vi "UpdatePanels.vi"(8 "error in (no error)":errorcluster, 10 "Engine in":refnum<class "Engine.lvclass">, 11 "BounceDemo in":refnum<class "BounceDemo.lvclass">) -> (0 "error out":errorcluster, 2 "Engine out":refnum<class "Engine.lvclass">, 3 "Game out":refnum<class "BounceDemo.lvclass">)   [LabVIEW 2019, in "RT_Game.lvlib" / "BounceDemo.lvclass"]
uses:
  BounceDemo.lvclass
  C:/Users/FreshBob/Dropbox/VIs/myRIO_GameConsole/RT/RT_Game/Bouncer/Bouncer.lvclass
  Engine/Engine.lvclass
  Bouncer/Bouncer.lvclass/Bouncer.ctl
  Bouncer/Read Panel1.vi
  Bouncer/Read Panel2.vi
  Bouncer/Read Ball.vi
  Bouncer/Write Panel1.vi
  Bouncer/Write Panel2.vi
  BouncePanel/BouncePanel.lvclass
  PongBall/PongBall.lvclass
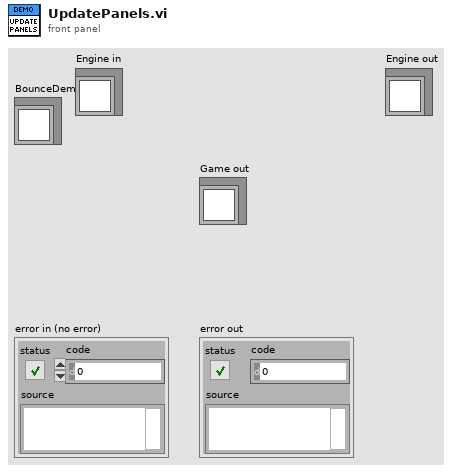
[diagram p1: front panel]
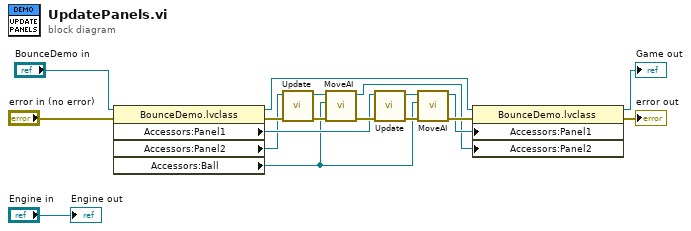
[diagram p0: block diagram]
diagram:
  n1 = property class="BounceDemo.lvclass"(reference="BounceDemo in", error in="error in (no error)") -> (reference out=w9:refnum<class "BounceDemo.lvclass">, error out=w15:errorcluster, "Accessors:Panel1"=w12:refnum<class "BouncePanel.lvclass">, "Accessors:Panel2"=w11:refnum<class "BouncePanel.lvclass">, "Accessors:Ball"=w4:refnum<class "PongBall.lvclass">)
  n2 = call-dynamic "Update.vi"("error in (no error)"=w15, "GameObject in"=w11) -> ("error out"=w6:errorcluster, "GameObject out"=w5:refnum<class "BouncePanel.lvclass">)  [unwired: 8 in]
  n3 = call-dynamic "MoveAI.vi"("error in (no error)"=w6, "Ball"=w4, "BouncePanel in"=w5) -> ("error out"=w16:errorcluster, "BouncePanel out"=w7:refnum<class "BouncePanel.lvclass">)  [unwired: 7 in]
  n4 = call-dynamic "Update.vi"("error in (no error)"=w16, "GameObject in"=w12) -> ("error out"=w18:errorcluster, "GameObject out"=w17:refnum<class "BouncePanel.lvclass">)  [unwired: 8 in]
  n5 = call-dynamic "MoveAI.vi"("error in (no error)"=w18, "Ball"=w4, "BouncePanel in"=w17) -> ("error out"=w10:errorcluster, "BouncePanel out"=w8:refnum<class "BouncePanel.lvclass">)  [unwired: 7 in]
  n6 = property class="BounceDemo.lvclass"(reference=w9, error in=w10, "Accessors:Panel1"=w8, "Accessors:Panel2"=w7) -> (reference out=→"Game out":refnum<class "BounceDemo.lvclass">, error out=→"error out":errorcluster)
  "Engine out" <- "Engine in"
